vi "例7-5(2).vi"() -> ()   [LabVIEW 2019]
panel:
  in  "停止按钮":bool
  out "告警":bool
  out "闸门开启高度(m)":dbl(slide) scale=0.0..10.0
  out "水流量(m^3/s)":dbl(knob) scale=0.0..30.0
  out "水位(m)":dbl(slide) scale=0.0..30.0
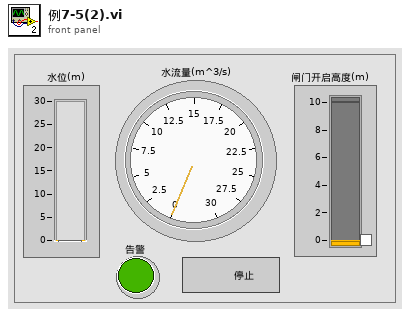
[diagram p1: front panel]
types:
  T1 = enum16{"Read", "Write", "ReadWrite", "BufferedRead", "BufferedReadWrite"}
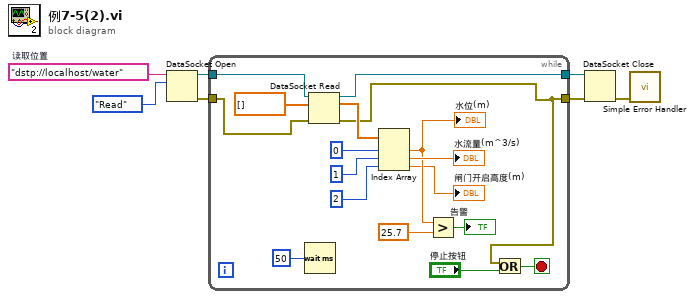
[diagram p0: block diagram]
diagram:
  w6 = "dstp://localhost/water"  # 读取位置
  n1 = DataSocket Open(10:T1."Read" ("模式"), 11:w6) -> (0:w4:errorcluster, 3:w5:refnum<k13>)  [unwired: 2 in]
  n2 = while {
    tunnel: w5 -> [w13]
    tunnel: w4 -> [w12]
    tunnel: [w11] -> w3
    tunnel: [w8] -> w2
    stop <- w9 stop-if-true
    n3 = Wait (ms)(milliseconds to wait=50) -> ()  [unwired: 1 out]
    n4 = DataSocket Read(8:w12, 10:dbl[] [], 11:w13) -> (0:w8:errorcluster, 2:w23:dbl[], 3:w11:refnum<k13>)  [unwired: 2 in, 4 out]
    n5 = Index Array(array=w23, index #1=0, index #2=1, index #3=2) -> (element #1=w17:dbl, element #2=→"水流量(m^3/s)":dbl, element #3=→"闸门开启高度(m)":dbl)
    "水位(m)" <- w17
    n6 = Greater?(x=w17, y=25.7) -> (0:→"告警":bool)
    n7 = Or(x=w8, y="停止按钮") -> (x .or. y?=w9:bool)
  }
  n8 = DataSocket Close(8:w2, 11:w3) -> (0:w1:errorcluster)  [unwired: 1 in, 1 out]
  n9 = call <vilib>:"Simple Error Handler.vi"("error in (no error)"=w1) -> ()  [unwired: 4 in, 5 out]
